vi "Get Device Name.vi"(8 "error in (no error)":errorcluster, 10 "DeviceIndex":u32, 11 "RTL-SDR in":refnum<class "RTL-SDR.lvclass">) -> (0 "error out":errorcluster, 2 "Device Name":string, 3 "RTL-SDR out":refnum<class "RTL-SDR.lvclass">)   [LabVIEW 2015, in "RTL-SDR.lvclass"]
uses:
  RTL-SDR.lvclass
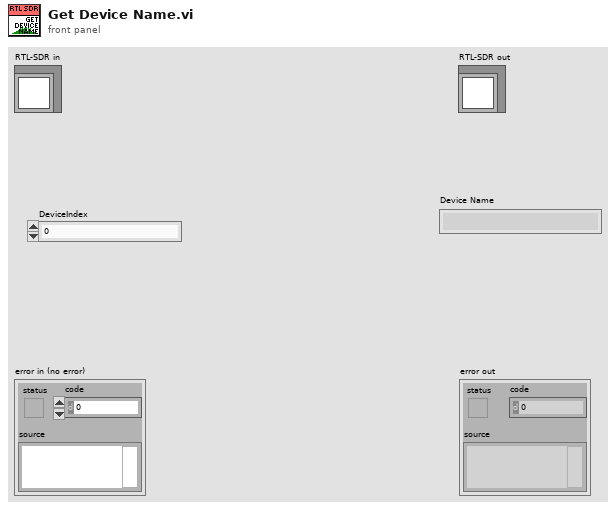
[diagram p1: front panel]
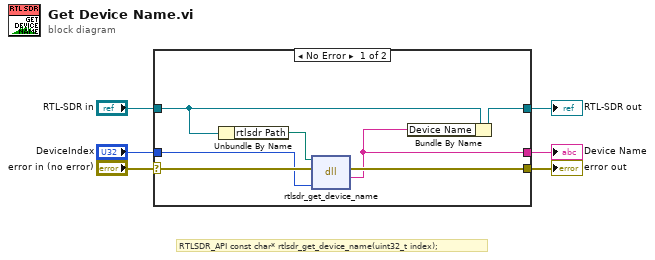
[diagram p0: block diagram]
diagram:
  # "RTLSDR_API const char* rtlsdr_get_device_name(uint32_t index);"
  n1 = case shown="No Error" "error in (no error)" {
    selector: "error in (no error)" -> [w13 w15]
    tunnel: [w12 w15] -> w5
    tunnel: [w8 w14] -> w3
    tunnel: "RTL-SDR in" -> [w11 w14]
    tunnel: "DeviceIndex" -> [w9 _]
    tunnel: [w7 _] -> w1
    frame No Error {
      n2 = Unbundle By Name(w11) -> ("rtlsdr Path"=w10:path)
      n3 = dll-call lib="C:/Users/Ivan/Desktop/D-23-09-24 (RTL-SDR)/Project (Pelleng-SDR)/rtlsdr/dll/rtlsdr.*" fn="rtlsdr_get_device_name"(path in=w10, error in=w13, "index"=w9) -> (error out=w12:errorcluster, "return type"=w7:string)  [unwired: 2 in, 1 out]
      n4 = Bundle By Name(cluster=w11, "Device Name"=w7) -> (w8:refnum<class "RTL-SDR.lvclass">)
    }
    frame Error {
    }
  }
  "error out" <- w5
  "RTL-SDR out" <- w3
  "Device Name" <- w1
